vi "RemoveErrorCameras.vi"(6 "error text":string[](array[string]), 8 "error in (no error)":errorcluster, 10 "error cameras":T1[](array[typedef]), 11 "Qbus in":refnum<class "Qbus.lvclass">) -> (0 "error out":errorcluster)   [LabVIEW 2017, in "IrAcquisition.lvlib"]
uses:
  <vilib>/addons/InsightCM/Devices/Shared/Ir/IrAcquisition/IrAcquisition.lvlib
  <vilib>/addons/InsightCM/Devices/Shared/Ir/IrAcquisition/controls/camera.ctl
  <vilib>/userdefined/High Color/IMAQdx.ctl
  <vilib>/vision/Image Controls.llb/IMAQ Image.ctl
  <vilib>/addons/PointValueMap/controls/PointMap.ctl
  <vilib>/addons/Qbus/Qbus.lvclass
  <vilib>/addons/InsightCM/Devices/Shared/Ir/IrManageCameras/IrManageCameras.lvlib
  <vilib>/addons/PointValueMap/PointValueMap.lvlib
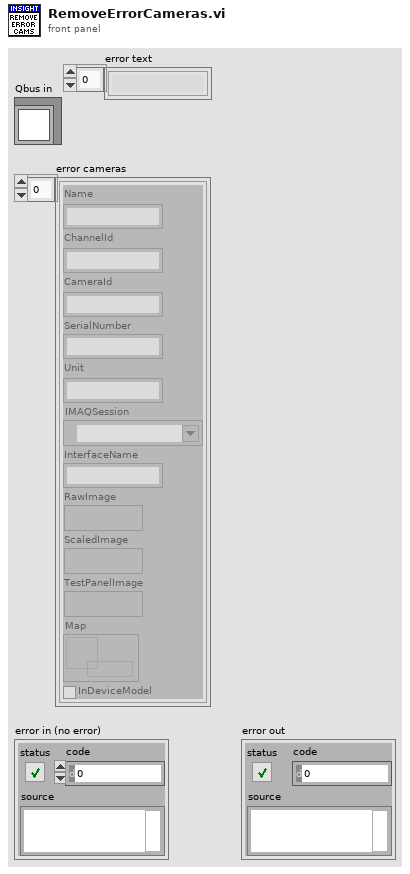
[diagram p1: front panel]
types:
  T1 = typedef "IrAcquisition.lvlib/camera.ctl" = cluster{"Name":string, "ChannelId":string, "CameraId":string, "SerialNumber":string, "Unit":string, "IMAQSession":T2, "InterfaceName":string, "RawImage":T3, "ScaledImage":T3, "TestPanelImage":T3, "Map":T4, "InDeviceModel":bool}
  T2 = typedef "IMAQdx.ctl" = refnum<k21>
  T3 = typedef "IMAQ Image.ctl" = refnum<image>
  T4 = typedef "PointValueMap.lvlib/PointMap.ctl" = refnum<data-value>
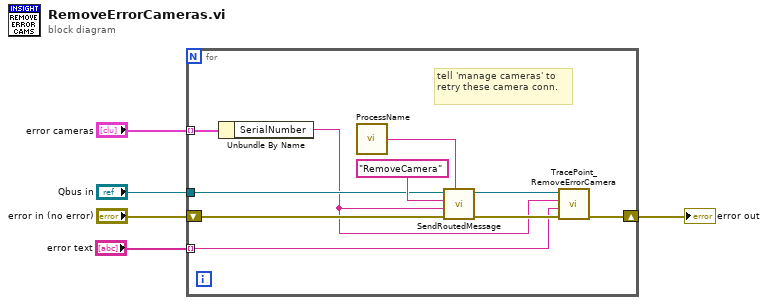
[diagram p0: block diagram]
diagram:
  n1 = for {
    tunnel: "error cameras" -> [w15] mode=indexing
    tunnel: "Qbus in" -> [w11]
    shift-right: [w9] -> w4
    shift-left: "error in (no error)" -> [w12]
    tunnel: "error text" -> [w6] mode=indexing
    # "tell 'manage cameras' to retry these camera conn."
    n2 = Unbundle By Name(w15) -> ("SerialNumber"=w7:string)
    n3 = call <vilib>:"ProcessName.vi"() -> ("process name"=w14:string)  [unwired: 5 in]
    n4 = call <vilib>:"SendRoutedMessage.vi"("listener process"=w14, "error in (no error)"=w12, "message value"=w7, "message name"="RemoveCamera", "Qbus in"=w11) -> ("error in (no error)"=w10:errorcluster, "Qbus out"=w8:refnum<class "Qbus.lvclass">)  [unwired: 5 in]
    n5 = call <vilib>:"TracePoint_RemoveErrorCamera.vi"("error in (no error)"=w10, "error text"=w6, "serial number"=w7, "Qbus"=w8) -> ("error out"=w9:errorcluster)  [unwired: 7 in]
  }
  "error out" <- w4
